vi "Status.vi"(8 "error in (no error)":errorcluster, 11 "Git Updater Module in":refnum<class "Git Updater Module.lvclass">) -> (0 "error out":errorcluster, 3 "Git Updater Module out":refnum<class "Git Updater Module.lvclass">)   [LabVIEW 2020, in "VolatusGUI.lvlib" / "Git Updater Module.lvclass"]
uses:
  Git Updater Module.lvclass
  <vilib>/Hampel Software Engineering/Git API/Git API/GIT-api.lvclass/GIT-api.ctl
  Git Updater Module.lvclass/Git Updater Module.ctl
  <vilib>/Hampel Software Engineering/Git API/Git API/GIT-api.lvclass
  Status.ctl
  Path Status.ctl
panel:
  out "Path Statuses":T1[](array[typedef])
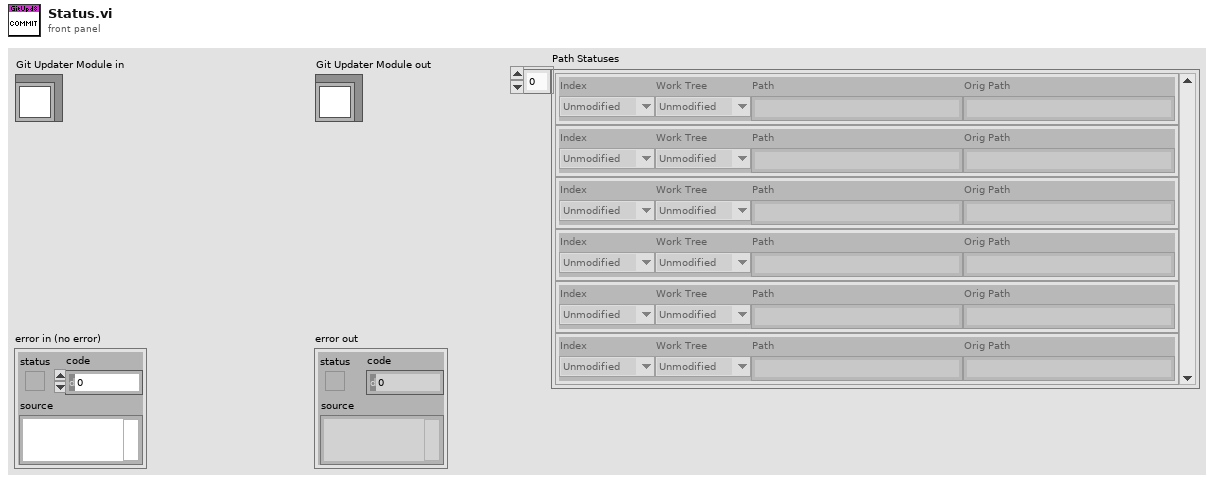
[diagram p1: front panel]
types:
  T1 = typedef "VolatusGUI.lvlib/Git Updater Module.lvclass/Path Status.ctl" = cluster{"Index":T2, "Work Tree":T2, "Path":string, "Orig Path":string}
  T2 = typedef "VolatusGUI.lvlib/Git Updater Module.lvclass/Status.ctl" = enum16{"UNKNOWN", "Unmodified", "Modified", "Added", "Deleted", "Renamed", "Unmerged", "Untracked", "Ignored"}
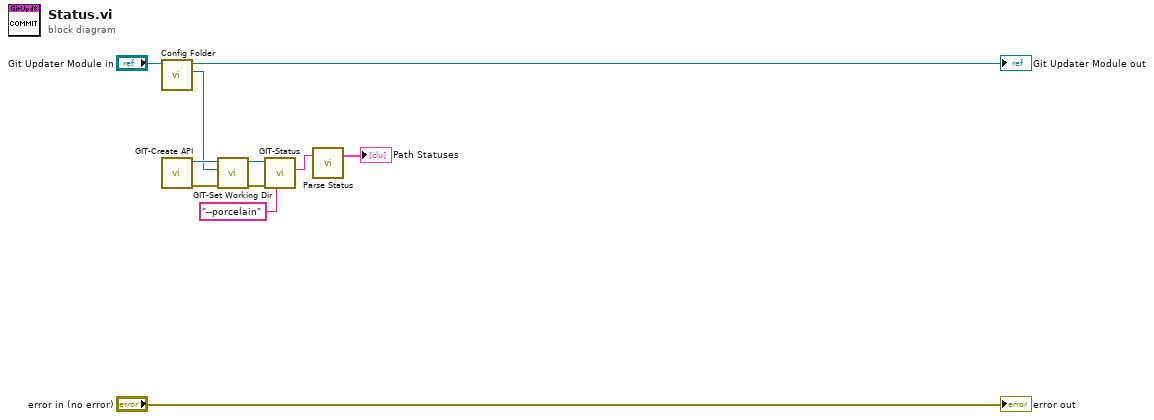
[diagram p0: block diagram]
diagram:
  n1 = call "Config Folder.vi"("Git Updater Module in"="Git Updater Module in") -> ("Config Folder"=w1:path, "Git Updater Module out"=→"Git Updater Module out":refnum<class "Git Updater Module.lvclass">)  [unwired: 8 in, 1 out]
  n2 = call <vilib>:"GIT-Create API.vi"() -> ("error out"=w8:errorcluster, "git-api out"=w7:refnum<class "GIT-api.lvclass">)  [unwired: 10 in]
  n3 = call <vilib>:"GIT-Set Working Dir.vi"("error in"=w8, "Working Directory"=w1, "git-api in"=w7) -> ("error out"=w5:errorcluster, "git-api out"=w6:refnum<class "GIT-api.lvclass">)  [unwired: 7 in]
  n4 = call <vilib>:"GIT-Status.vi"("param"="--porcelain", "error in"=w5, "git-api in"=w6) -> ("std out"=w3:string)  [unwired: 6 in, 2 out]
  n5 = call "Parse Status.vi"("Status"=w3) -> ("Path Statuses"=→"Path Statuses":T1[])  [unwired: 6 in]
  "error out" <- "error in (no error)"
